vi "Calc Block Width.vi"(11 "State In":T1) -> (3 "State":T1)   [LabVIEW 2020, in "FlexBlock.xnode"]
uses:
  FlexBlock.xnode
  State.ctl
  FlexBlocks/Type Descriptor.ctl
  FlexBlocks/Terminal Direction.ctl
  FlexBlocks/Value Mode.ctl
  FlexBlocks/Terminal State.ctl
  FlexBlocks/Special Terminal.ctl
  FlexBlocks/Errors.ctl
  <vilib>/picture/picture.llb/imagedata.ctl
  FlexBlocks/Calculated Sizes.ctl
  FlexBlocks/FlexBlocks.lvlib
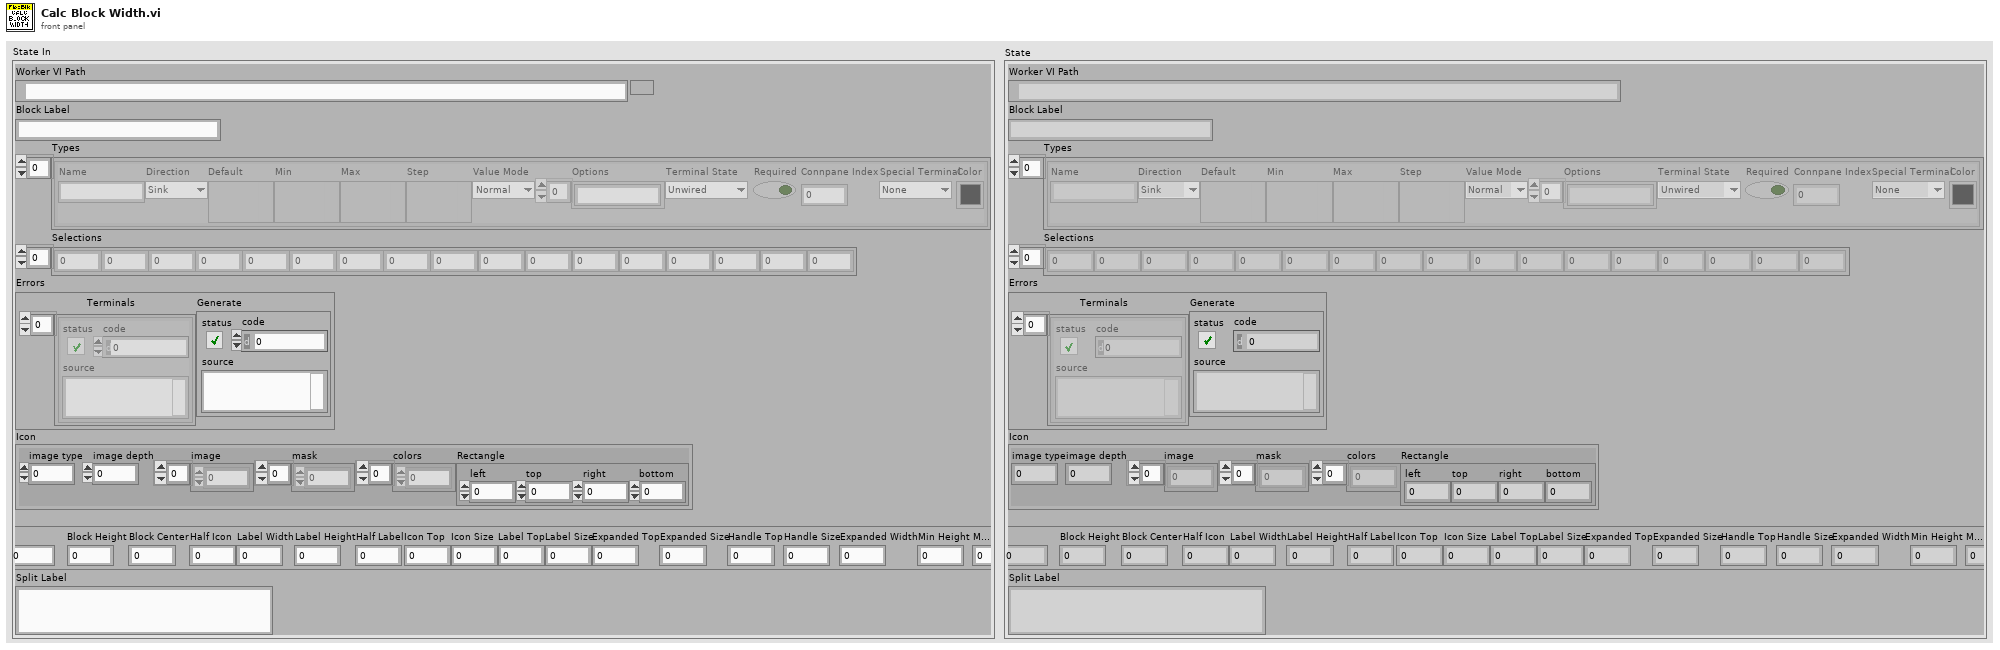
[diagram p1: front panel]
types:
  T1 = typedef "FlexBlock.xnode/State.ctl" = cluster{"Worker VI Path":path, "Block Label":string, "Types":T2[], "Selections":i32[], "Errors":T7, "Icon":T8, "Calcd Sizes":T9, "Split Label":string}
  T2 = typedef "FlexBlocks.lvlib/Type Descriptor.ctl" = cluster{"Name":string, "Direction":T3, "Default":variant, "Min":variant, "Max":variant, "Step":variant, "Value Mode":T4, "Options":string[], "Terminal State":T5, "Required":bool, "Connpane Index":i32, "Special Terminal":T6, "Color":u32}
  T3 = typedef "FlexBlocks.lvlib/Terminal Direction.ctl" = enum16{"Sink", "Source"}
  T4 = typedef "FlexBlocks.lvlib/Value Mode.ctl" = enum16{"Normal", "Range", "Select"}
  T5 = typedef "FlexBlocks.lvlib/Terminal State.ctl" = enum16{"Unwired", "BadType", "BadRef", "Channel", "Value", "Control Ref"}
  T6 = typedef "FlexBlocks.lvlib/Special Terminal.ctl" = enum16{"None", "Action", "Init", "Tag", "State in", "State out", "Error"}
  T7 = typedef "FlexBlocks.lvlib/Errors.ctl" = cluster{"Terminals":errorcluster[], "Generate":errorcluster}
  T8 = typedef "imagedata.ctl" = cluster{"image type":i32, "image depth":i32, "image":u8[], "mask":u8[], "colors":u32[], "Rectangle":cluster{"left":i16, "top":i16, "right":i16, "bottom":i16}}
  T9 = typedef "FlexBlocks.lvlib/Calculated Sizes.ctl" = cluster{"Text Width":i32, "Text Height":i32, "Half Text":i32, "Block Width":i32, "Block Height":i32, "Block Center":i32, "Half Icon":i32, "Label Width":i32, "Label Height":i32, "Half Label":i32, "Icon Top":i32, "Icon Size":i32, "Label Top":i32, "Label Size":i32, "Expanded Top":i32, "Expanded Size":i32, "Handle Top":i32, "Handle Size":i32, "Expanded Width":i32, "Min Height":i32, "Max Height":i32}
  T10 = typedef "FlexBlocks.lvlib/Size Constants.ctl" = cluster{"Icon":i32, "Value Width":i32, "BG Rounding":i32, "Term Width":i32, "Term Height":i32, "Text Offset":i32, "Value Padding":i32, "Select Padding":i32, "Min Block Width":i32, "Vertical Margin":i32, "Size Handle Height":i32, "Name Padding":i32}
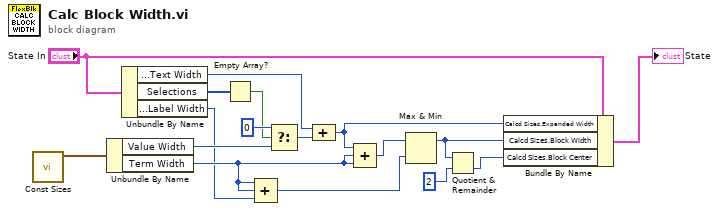
[diagram p0: block diagram]
diagram:
  n1 = call "Const Sizes.vi"() -> ("Sizes"=w17:T10)  [unwired: 11 in]
  n2 = Unbundle By Name(w17) -> ("Value Width"=w12:i32, "Term Width"=w3:i32)
  n3 = Unbundle By Name("State In") -> ("Calcd Sizes.Text Width"=w16:i32, "Selections"=w13:i32[], "Calcd Sizes.Label Width"=w2:i32)
  n4 = Empty Array?(array=w13) -> (empty?=w9:bool)
  n5 = Compound Arithmetic op=ADD(w3, w3, w2) -> (w1:i32)
  n6 = Select(t=0, s=w9, f=w12) -> (s? t:f=w11:i32)
  n7 = Compound Arithmetic op=ADD(w16, w11) -> (w5:i32)
  n8 = Compound Arithmetic op=ADD(w5, w3, w3) -> (w4:i32)
  n9 = Max & Min(x=w4, y=w1) -> (max(x,y)=w8:i32)  [unwired: 1 out]
  n10 = Quotient & Remainder(x=w8, y=2) -> (floor(x/y)=w6:i32)  [unwired: 1 out]
  n11 = Bundle By Name(cluster="State In", "Calcd Sizes.Expanded Width"=w5, "Calcd Sizes.Block Width"=w8, "Calcd Sizes.Block Center"=w6) -> (→"State":T1)
